vi "Test DeluxeWash.vi"(8 "error in (no error)":errorcluster, 11 "TestCase in":refnum<class "CarWashTestCases.lvclass">) -> (0 "error out":errorcluster, 3 "TestCase out":refnum<class "CarWashTestCases.lvclass">)   [LabVIEW 2018, in "CarWashTestCases.lvclass"]
uses:
  CarWashTestCases.lvclass
  Command.ctl
  <vilib>/addons/_JKI Toolkits/VI Tester/TestCase.llb/TestCase.lvclass
  C:/Program Files (x86)/National Instruments/LabVIEW 2018/vi.lib/addons/_JKI Toolkits/VI Tester/TestCase.llb/TestCase.lvclass
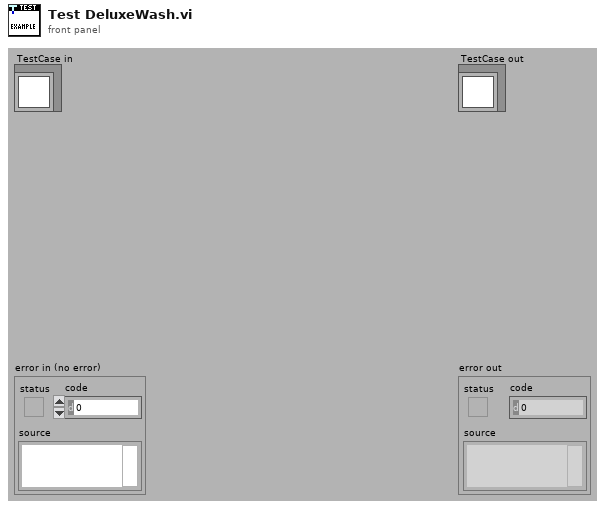
[diagram p1: front panel]
types:
  T1 = typedef "Command.ctl" = enum16{"Underbody Wash", "Soap Application", "Main High-Pressure Wash", "Clear Water Rinse", "Air Dry Cycle", "Stop"}
  T2 = typedef "MessageQueueData.ctl" = cluster{"State":T1, "Data":variant}
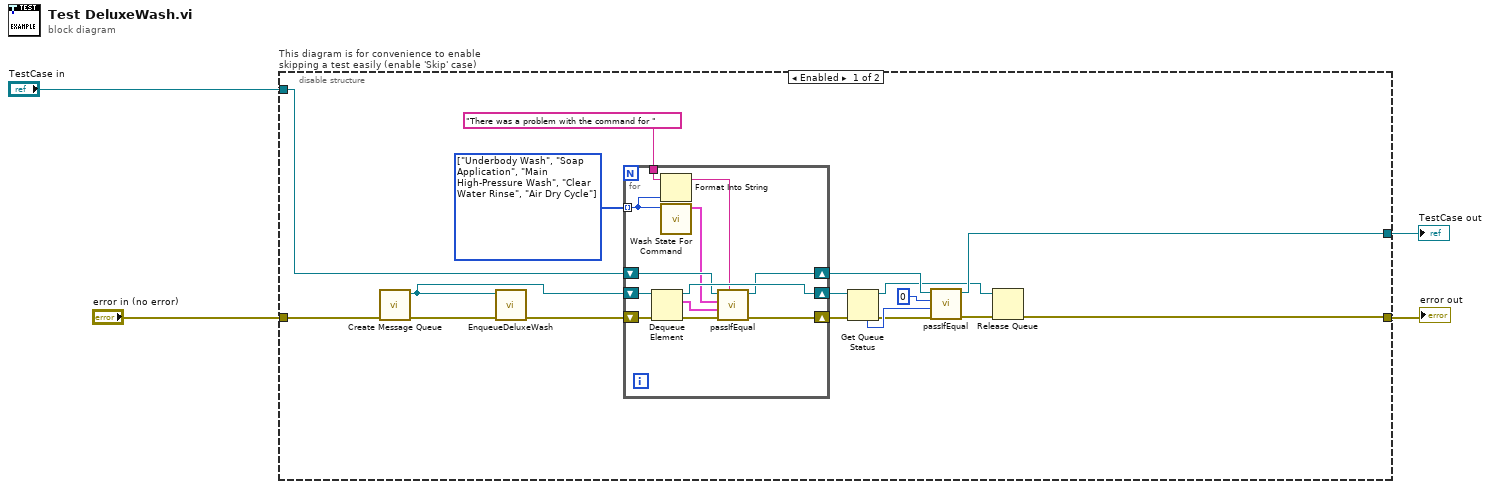
[diagram p0: block diagram]
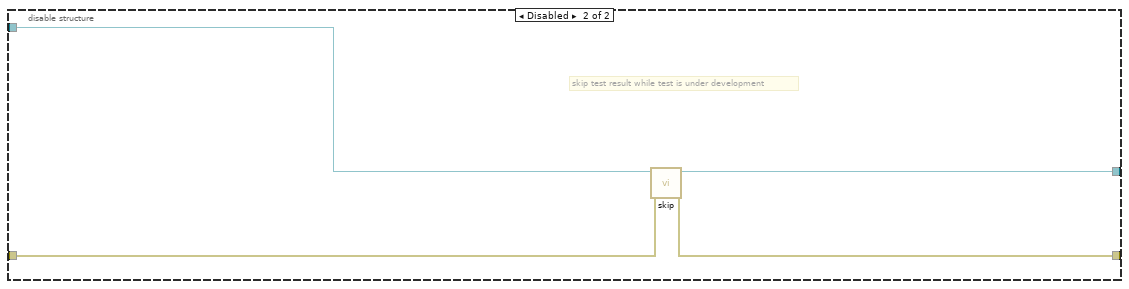
[diagram p2: hidden frame]
diagram:
  n1 = disable-structure "This diagram is for convenience to enable skipping a test easily (enable 'Skip' case)" shown="Enabled" {
    disable-tunnel: "TestCase in" -> [w15 w37]
    disable-tunnel: [w21 w35] -> w1
    disable-tunnel: [w8 w36] -> w3
    disable-tunnel: "error in (no error)" -> [w20 w34]
    frame Enabled {
      w16 = T1[] [enum."Underbody Wash", enum."Soap Application", enum."Main High-Pressure Wash", enum."Clear Water Rinse", enum."Air Dry Cycle"] items=["Underbody Wash", "Soap Application", "Main High-Pressure Wash", "Clear Water Rinse", "Air Dry Cycle", "Stop"]
      n2 = call "Create Message Queue.vi"("error in (no error)"=w20) -> ("error out"=w19:errorcluster, "Queue out"=w17:refnum<queue>)  [unwired: 9 in]
      n3 = call "EnqueueDeluxeWash.vi"("error in (no error)"=w19, "Queue in"=w17) -> ("error out"=w18:errorcluster)  [unwired: 9 in]
      n4 = for {
        shift-right: [w32] -> w12
        shift-left: w17 -> [w31]
        shift-right: [w29] -> w13
        shift-left: w18 -> [w33]
        tunnel: w16 -> [w26] mode=indexing
        shift-right: [w27] -> w6
        shift-left: w15 -> [w28]
        tunnel: "There was a problem with the command for " ("custom report message (\"\")") -> [w25]
        n5 = Dequeue Element(queue=w31, error in (no error)=w33) -> (queue out=w32:refnum<queue>, element=w22:T2, error out=w30:errorcluster)  [unwired: 1 in, 1 out]
        n6 = Format Into String(initial string=w25, w26) -> (resulting string=w24:string)  [unwired: 2 in, 1 out]
        n7 = call "Wash State For Command.vi"("Command"=w26) -> ("Queue Data for Command"=w23:T2)  [unwired: 10 in]
        n8 = call-dynamic "passIfEqual.vi"("custom report message (\"\")"=w24, "error in (no error)"=w30, "y"=w22, "x"=w23, "TestCase in"=w28) -> ("error out"=w29:errorcluster, "TestCase out"=w27:refnum<class "CarWashTestCases.lvclass">)  [unwired: 5 in]
      }
      n9 = Get Queue Status(queue=w12, error in (no error)=w13) -> (queue out=w5:refnum<queue>, error out=w7:errorcluster, # elements in queue=w11:i32)  [unwired: 1 in, 5 out]
      n10 = call-dynamic "passIfEqual.vi"("error in (no error)"=w7, "y"=w11, "x"=0 ("# elements in queue"), "TestCase in"=w6) -> ("error out"=w9:errorcluster, "TestCase out"=w21:refnum<class "CarWashTestCases.lvclass">)  [unwired: 6 in]
      n11 = Release Queue(queue=w5, error in (no error)=w9) -> (error out=w8:errorcluster)  [unwired: 1 in, 2 out]
    }
    frame Disabled {
      # "skip test result while test is under development"
      n12 = call <vilib>:"skip.vi"("error in (no error)"=w34, "TestCase in"=w37) -> ("error out"=w36:errorcluster, "TestCase out"=w35:refnum<class "CarWashTestCases.lvclass">)  [unwired: 8 in]
    }
  }
  "error out" <- w3
  "TestCase out" <- w1
